vi "test_shitty.vi"   [LabVIEW 2018]
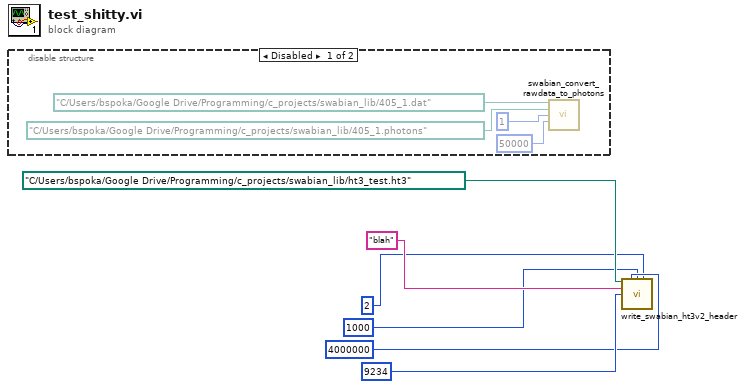
[diagram p0: block diagram]
diagram:
  n1 = disable-structure shown="Disabled" {
    frame Disabled {
      n2 = call "swabian_convert_rawdata_to_photons.vi"("Raw_data_file"=path "C:/Users/bspoka/Google Drive/Programming/c_projects/swabian_lib/405_1.dat" ("file path (use dialog)"), "output_data_file"=path "C:/Users/bspoka/Google Drive/Programming/c_projects/swabian_lib/405_1.photons" ("file path (use dialog)"), "sync_channel"=1, "sync_period_ps"=u64 50000 ("sync_rate")) -> ()  [unwired: 11 in, 1 out]
    }
    frame Enabled {
    }
  }
  n3 = call "write_swabian_ht3v2_header.vi"("data_path"=path "C:/Users/bspoka/Google Drive/Programming/c_projects/swabian_lib/ht3_test.ht3", "acq_time"=4000000 ("acq_mode"), "sync_rate"=1000, "acq_mode"=2 ("acq_time"), "data_comment"="blah", "num_records"=u64 9234) -> ()  [unwired: 9 in, 1 out]
